vi "DEV Erase User Data.vi"(11 "DevHandle":i32) -> (3 "function return":bool)   [LabVIEW 2010, in "usb_device.lvlib"]
doc: "bool WINAPI DEV_EraseUserData(int DevHandle);"
uses:
  usb_device.lvlib
  USB2XXX.dll
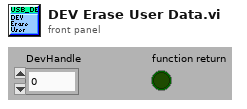
[diagram p1: front panel]
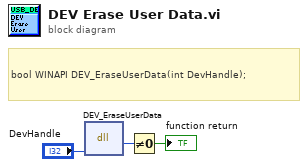
[diagram p0: block diagram]
diagram:
  # "bool WINAPI DEV_EraseUserData(int DevHandle);"
  n1 = dll-call lib="G:/OtherWork/USB2XXX_Example/trunk/Labview/PublicFiles/usb_device/USB2XXX.*" fn="DEV_EraseUserData"("DevHandle"="DevHandle") -> (w2:u8)  [unwired: 4 in, 2 out]
  n2 = Not Equal To 0?(x=w2) -> (x != 0?=→"function return":bool)
